vi "SVM_SWLDA_Calculator.vi"(5 "ERP_all_icon":dbl[][](array[numeric]) format="%0.3f", 7 "ModelFileName":string="C:\\\\WORK\\\\RBFModel", 8 "Target_total2 (from offline file)":path=path "C:/Users/Jaehong/Desktop/안전복지프로젝트/LabVIEW/RSVP_offline_onine/분석데이터/전선미_RSVP_Offline_Analysis2/2014-09-01/Target_Total2.txt", 9 "SWLDA_Weight":path=path "C:/Users/Jaehong/Desktop/안전복지프로젝트/LabVIEW/RSVP_offline_onine/분석데이터/전선미_RSVP_Offline_Analysis2/2014-09-01/Target_Total2.txt", 11 "ERP_Parameters_of_Target_prior.txt":path=path "C:/Users/Jaehong/Desktop/안전복지프로젝트/LabVIEW/RSVP_offline_onine/분석데이터/전선미_RSVP_Training_Test(LDA)/2014-08-29/ERP_Parameters_of_Target_prior.txt") -> (1 "ACC1(%)":dbl, 3 "Accuracy2(%)":dbl)   [LabVIEW 2013]
uses:
  <vilib>/Utility/file.llb/Read From Spreadsheet File (I64).vi
  <vilib>/Utility/file.llb/Read From Spreadsheet File (DBL).vi
panel:
  out "selected_all":i16[](array[numeric])
  out "test predict":dbl[](array[numeric])=[-1.0, -1.0, -1.0, -1.0, -1.0, -1.0, -1.0, -1.0, -1.0, -1.0, -1.0, -1.0, -1.0, -1.0, -1.0, -1.0, -1.0, -1.0, -1.0, -1.0, -1.0, -1.0, -1.0, -1.0, 1.0, -1.0, 1.0, 1.0, -1.0, 1.0, -1.0, -1.0, -1.0, -1.0, -1.0, -1.0, 1.0, -1.0, 1.0, -1.0, 1.0, -1.0, -1.0, -1.0]
  out "Squared correlation\n coefficient":dbl
  out "Total":i32
  out "correct":i16
  # "Results"
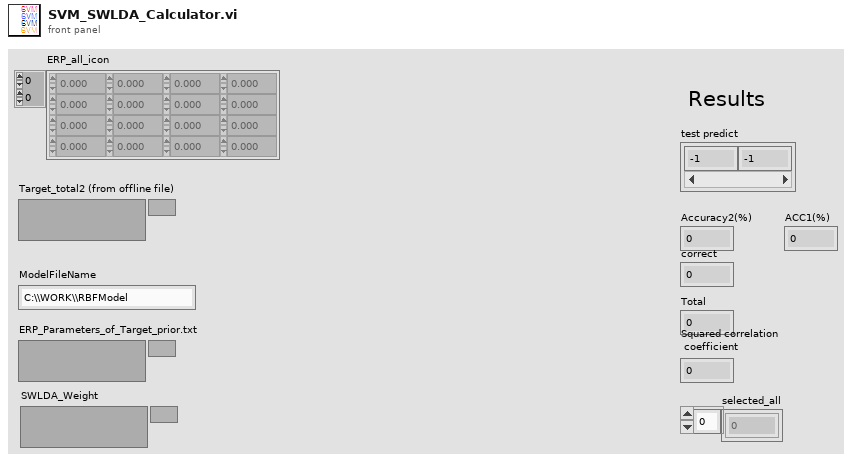
[diagram p1: front panel]
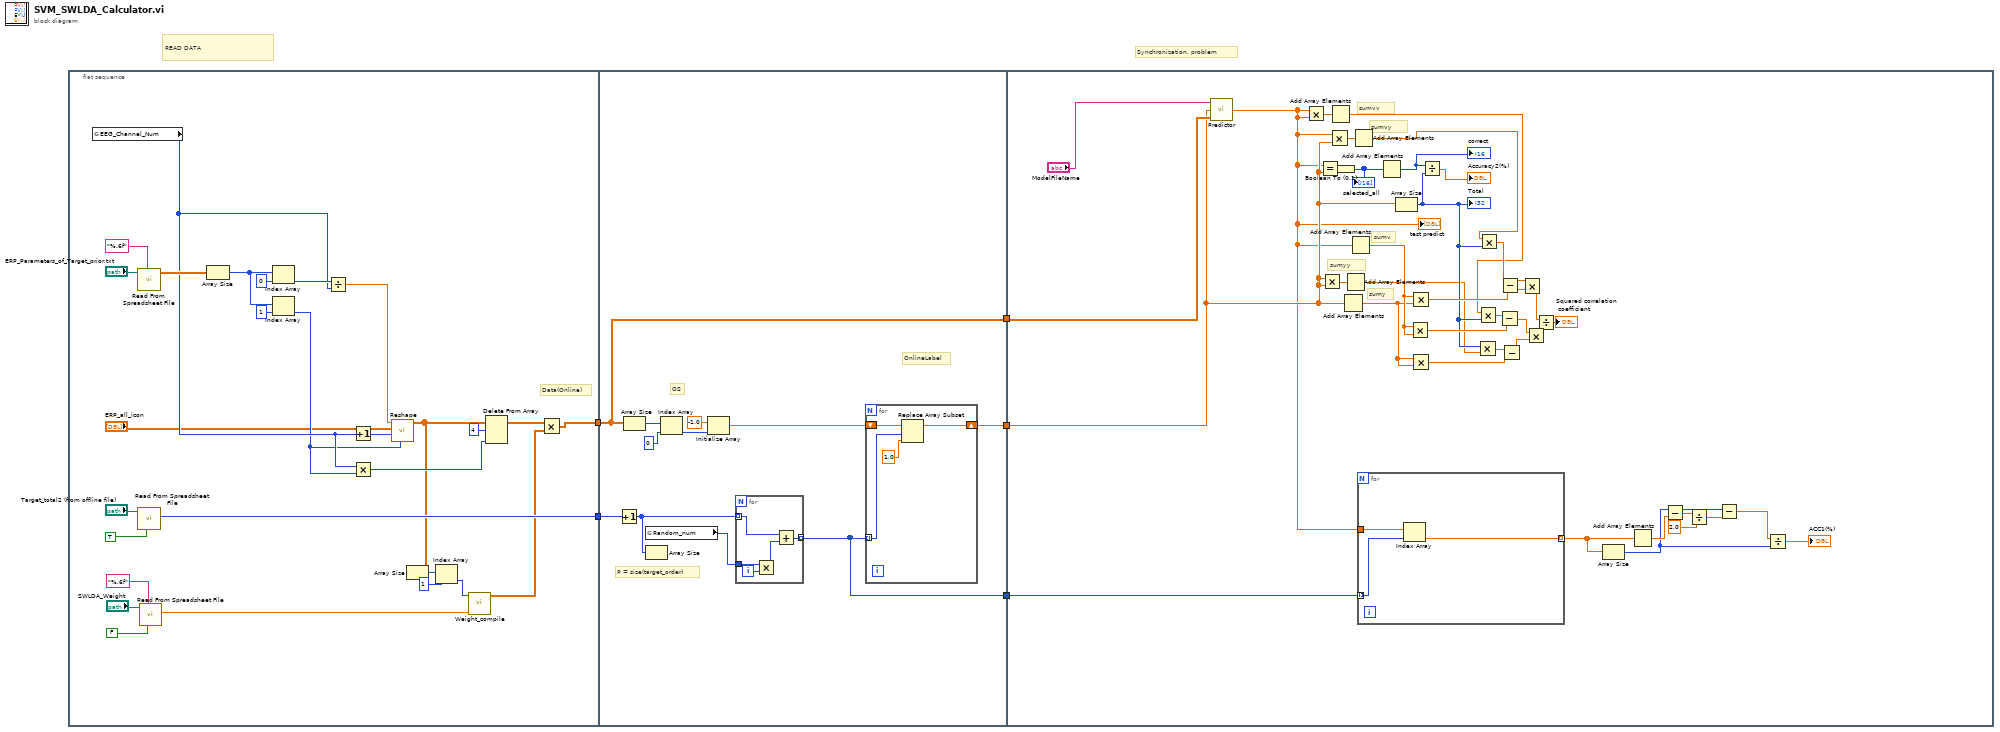
[diagram p0: block diagram]
diagram:
  # "Synchronization. problem"
  # "READ DATA"
  n1 = flat-sequence {
    tunnel: [w6] -> w5
    tunnel: [w29] -> w4
    tunnel: w5 -> [w35]
    tunnel: w4 -> [w42]
    tunnel: [w36] -> w3
    tunnel: [w35] -> w2
    tunnel: [w34] -> w1
    tunnel: w3 -> [w65]
    tunnel: w2 -> [w90]
    tunnel: w1 -> [w64]
    frame #0 {
      # "Data(Online)"
      n2 = global read "Control_Panel.vi" "EEG_Channel_Num"() -> (w19:i32)
      n3 = call-poly <vilib>:"Read From Spreadsheet File.vi"("format (%.3f)"="%.6f", "file path (dialog if empty)"="ERP_Parameters_of_Target_prior.txt") -> ("all rows"=w24:dbl[][])  [unwired: 5 in, 4 out]
      n4 = call-poly <vilib>:"Read From Spreadsheet File.vi"("transpose (no:F)"=TRUE, "file path (dialog if empty)"="Target_total2 (from offline file)") -> ("first row"=w29:i64[])  [unwired: 5 in, 4 out]
      n5 = call-poly <vilib>:"Read From Spreadsheet File.vi"("transpose (no:F)"=FALSE, "format (%.3f)"="%.6f", "file path (dialog if empty)"="SWLDA_Weight") -> ("first row"=w7:dbl[])  [unwired: 4 in, 4 out]
      n6 = Array Size(array=w24) -> (size(s)=w21:i32[])
      n7 = Index Array(array=w21, index=0) -> (element=w20:i32)
      n8 = Index Array(array=w21, index=1) -> (element=w17:i32)
      n9 = Divide(x=w20, y=w19) -> (x/y=w18:dbl)
      n10 = Increment(x=w19) -> (x+1=w31:i32)
      n11 = Multiply(x=w19, y=w17) -> (x*y=w27:i32)
      n12 = call "Reshape.vi"("Numeric"=w17, "EEG_Channel_Num"=w31, "all rows"="ERP_all_icon", "Numeric 2"=w18) -> ("Array"=w12:dbl[][])  [unwired: 7 in]
      n13 = Array Size(array=w12) -> (size(s)=w15:i32[])
      n14 = Index Array(array=w15, index=1) -> (element=w13:i32)
      n15 = call "Weight_compile.vi"("WEIGHT"=w7, "column_number"=w13) -> ("Compiled_weight"=w11:dbl[][])  [unwired: 9 in]
      n16 = Delete From Array(array=w12, length=4, index (col)=w27) -> (array with subset deleted=w30:dbl[][])  [unwired: 1 in, 1 out]
      n17 = Multiply(x=w30, y=w11) -> (x*y=w6:dbl[][])
    }
    frame #1 {
      # "OnlineLabel"
      # "P = size(target_order)"
      # "OS"
      n18 = Increment(x=w42) -> (x+1=w41:i64[])
      n19 = Array Size(array=w35) -> (size(s)=w44:i32[])
      n20 = global read "Control_Panel.vi" "Random_num"() -> (w40:i32)
      n21 = Array Size(array=w41) -> ()  [unwired: 1 out]
      n22 = Index Array(array=w44, index=0) -> (element=w39:i32)
      n23 = Initialize Array(-1.0 ("element"), w39) -> (w37:dbl[])
      n24 = for {
        tunnel: w41 -> [w50] mode=indexing
        tunnel: w40 -> [w52]
        tunnel: [w49] -> w34 mode=indexing
        i -> [w53]
        n25 = Multiply(x=w52, y=w53) -> (x*y=w51:i32)
        n26 = Add(x=w50, y=w51) -> (x+y=w49:i64)
      }
      n27 = for {
        tunnel: w34 -> [w47] mode=indexing
        shift-right: [w45] -> w36
        shift-left: w37 -> [w48]
        n28 = Replace Array Subset(array=w48, new element=1.0 ("new element/subarray"), index=w47) -> (w45:dbl[])
      }
    }
    frame #2 {
      # "sumyy"
      # "sumvy"
      # "sumvv"
      # "sumy"
      # "sumv"
      n29 = call "Predictor.vi"("attributes"=w90, "Lables"=w65, "ModelFileName"="ModelFileName") -> ("predictedlevel"=w63:dbl[])
      "test predict" <- w63
      n30 = Multiply(x=w63, y=w63) -> (x*y=w73:dbl[])
      n31 = Equal?(x=w63, y=w65) -> (x = y?=w68:bool[])
      n32 = Multiply(x=w65, y=w65) -> (x*y=w72:dbl[])
      n33 = Multiply(x=w63, y=w65) -> (x*y=w74:dbl[])
      n34 = Add Array Elements(numeric array=w73) -> (sum=w70:dbl)
      n35 = Boolean To (0,1)(Boolean=w68) -> (0, 1=w69:i16[])
      "selected_all" <- w69
      n36 = Add Array Elements(numeric array=w65) -> (sum=w82:dbl)
      n37 = Add Array Elements(numeric array=w72) -> (sum=w67:dbl)
      n38 = Add Array Elements(numeric array=w63) -> (sum=w85:dbl)
      n39 = Add Array Elements(numeric array=w74) -> (sum=w71:dbl)
      n40 = for {
        tunnel: w64 -> [w93] mode=indexing
        tunnel: w63 -> [w94]
        tunnel: [w92] -> w54 mode=indexing
        n41 = Index Array(array=w94, index=w93) -> (element=w92:dbl)
      }
      n42 = Add Array Elements(numeric array=w69) -> (sum=w66:i16)
      "correct" <- w66
      n43 = Array Size(array=w65) -> (size(s)=w75:i32)
      "Total" <- w75
      n44 = Multiply(x=w85, y=w85) -> (x*y=w84:dbl)
      n45 = Multiply(x=w85, y=w82) -> (x*y=w88:dbl)
      n46 = Multiply(x=w82, y=w82) -> (x*y=w81:dbl)
      n47 = Divide(x=w66, y=w75) -> (x/y=→"Accuracy2(%)":dbl)
      n48 = Multiply(x=w75, y=w67) -> (x*y=w83:dbl)
      n49 = Multiply(x=w70, y=w75) -> (x*y=w86:dbl)
      n50 = Multiply(x=w71, y=w75) -> (x*y=w89:dbl)
      n51 = Subtract(x=w86, y=w84) -> (x-y=w80:dbl)
      n52 = Subtract(x=w89, y=w88) -> (x-y=w87:dbl)
      n53 = Subtract(x=w83, y=w81) -> (x-y=w79:dbl)
      n54 = Multiply(x=w87, y=w87) -> (x*y=w78:dbl)
      n55 = Multiply(x=w80, y=w79) -> (x*y=w77:dbl)
      n56 = Divide(x=w78, y=w77) -> (x/y=→"Squared correlation\n coefficient":dbl)
      n57 = Array Size(array=w54) -> (size(s)=w57:i32)
      n58 = Add Array Elements(numeric array=w54) -> (sum=w61:dbl)
      n59 = Subtract(x=w57, y=w61) -> (x-y=w60:dbl)
      n60 = Divide(x=w60, y=2.0) -> (x/y=w58:dbl)
      n61 = Subtract(x=w57, y=w58) -> (x-y=w56:dbl)
      n62 = Divide(x=w56, y=w57) -> (x/y=→"ACC1(%)":dbl)
    }
  }
